vi "Read outputs.vi"(8 "error in":errorcluster, 11 "shared memory module runtime":refnum<class "shared memory runtime.lvclass">) -> (0 "error out":errorcluster, 2 "outputs":T1[](array[typedef]), 3 "shared memory module runtime out":refnum<class "shared memory runtime.lvclass">)   [LabVIEW 2013, in "shared memory runtime.lvclass"]
doc: "***TODO***\n\n<B>Input Parameters</B>\n\n<B>error in</B> describes error conditions that occur before this node runs. This input provides standard error in functionality.\n\n<B>shared memory module runtime</B> ***TODO***shared memory module runtime\n\n<B>Output Parameters</B>\n\n<B>error out</B> contains error information. This output provides standard error out functionality.\n\n<B>outputs</B> ***TODO***outputs\n\n<B> * channel classification</B> ***TODO***outputs.channel classification***enum values: input data,output data,processing parameter,processing result\n\n<B> * data type</B> ***TODO***outputs.data type***enum values: Double,Single,I64,I32,I16,I8,U64,U32,U16,U8,Boolean,String,Array of Double,Array of Single,Array of I64,Array of I32,Array of I16,Array of I8,Array of U64,Array of U32,Array of U16,Array of U8,Array of Boolean,Array of String\n\n<B> * pointer to shared memory</B> ***TODO***outputs.pointer to shared memory\n\n<B> * number of elements</B> ***TODO***outputs.number of elements\n\n<B> * shared memory</B> ***TODO***outputs.shared memory\n\n<B> * data dictionary index</B> ***TODO***outputs.data dictionary index\n\n<B> * data dictionary index.</B> ***TODO***outputs.data dictionary index.\n\n<B>shared memory module runtime out</B> ***TODO***shared memory module runtime out"
uses:
  shared memory runtime.lvclass
  <vilib>/NI/Tag Bus/tag/Data Type.ctl
  <vilib>/NI/Tag Bus/tag/tag descriptor.lvclass
  shared memory module runtime.ctl
  <vilib>/NI/Tag Bus Module Framework/channel/channel classification.ctl
  <vilib>/NI/Tag Bus Module Framework/channel/TBM channel.lvclass
  <vilib>/National Instruments/Shared Memory Library for Linux RT/Classes/Shared Memory/Shared Memory.lvclass
  <vilib>/National Instruments/Shared Memory Library for Linux RT/Controls/Shared Memory Class Reference.ctl
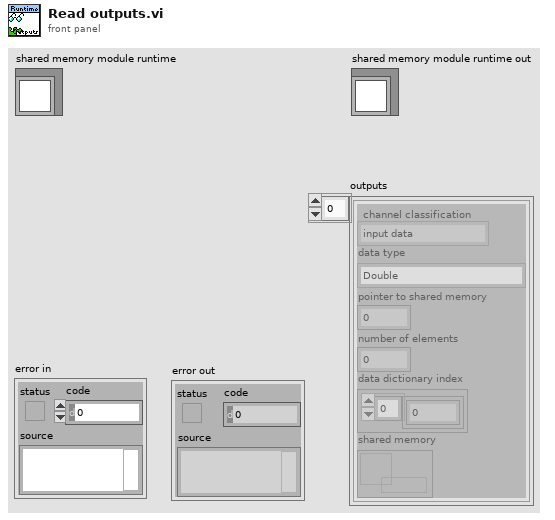
[diagram p1: front panel]
types:
  T1 = typedef "shared memory runtime.lvclass/shared memory module runtime.ctl" = cluster{"channel classification":T2, "data type":T3, "pointer to shared memory":u64, "number of elements":u64, "data dictionary index":cluster{i32[]}, "shared memory":T4}
  T2 = typedef "TBM channel.lvclass/channel classification.ctl" = enum16{"input data", "output data", "processing parameter", "processing result"}
  T3 = typedef "tag bus.lvlib/tag descriptor.lvclass/Data Type.ctl" = enum16{"Double", "Single", "I64", "I32", "I16", "I8", "U64", "U32", "U16", "U8", "Boolean", "String", "Array of Double", "Array of Single", "Array of I64", "Array of I32", "Array of I16", "Array of I8", "Array of U64", "Array of U32", "Array of U16", "Array of U8", "Array of Boolean", "Array of String"}
  T4 = typedef "Shared Memory Class Reference.ctl" = refnum<data-value>
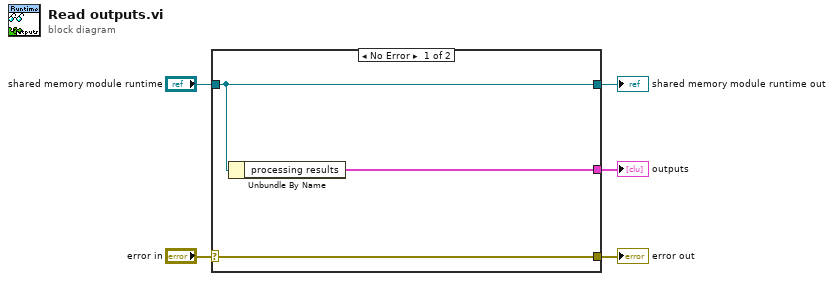
[diagram p0: block diagram]
diagram:
  n1 = case shown="No Error" "error in" {
    selector: "error in" -> [w8 w9]
    tunnel: [w8 w9] -> w4
    tunnel: [w7 w10] -> w2
    tunnel: "shared memory module runtime" -> [w7 w10]
    tunnel: [w6 _] -> w1
    frame No Error {
      n2 = Unbundle By Name(w7) -> ("processing results"=w6:T1[])
    }
    frame Error {
    }
  }
  "error out" <- w4
  "shared memory module runtime out" <- w2
  "outputs" <- w1
